vi "init.vi"(0 "Digital Input Test in":refnum<class "Set Motor Power Test.lvclass">, 1 "Command":u16, 2 "ConfigureILCStrategy":refnum<class "IConfigureILCStrategy.lvclass">, 5 "error in (no error)":errorcluster, 6 "Test Scenario":T1, 7 "Log":refnum<class "ITestLog.lvclass">, 8 "Signal Name":string) -> (14 "Digital Input Test out":refnum<class "Set Motor Power Test.lvclass">, 19 "error out":errorcluster)   [LabVIEW 2015, in "Set Motor Power Test.lvclass"]
uses:
  Set Motor Power Test.lvclass
  Model/TestLog/ITestLog/ITestLog.lvclass
  Typedefs/TestScenarioTypes.ctl
  Model/ConfigureILCStrategy/IConfigureILCStrategy/IConfigureILCStrategy.lvclass
  Set Motor Power Test.lvclass/Set Motor Power Test.ctl
  Typedefs/ILCBTTypedefs.lvlib
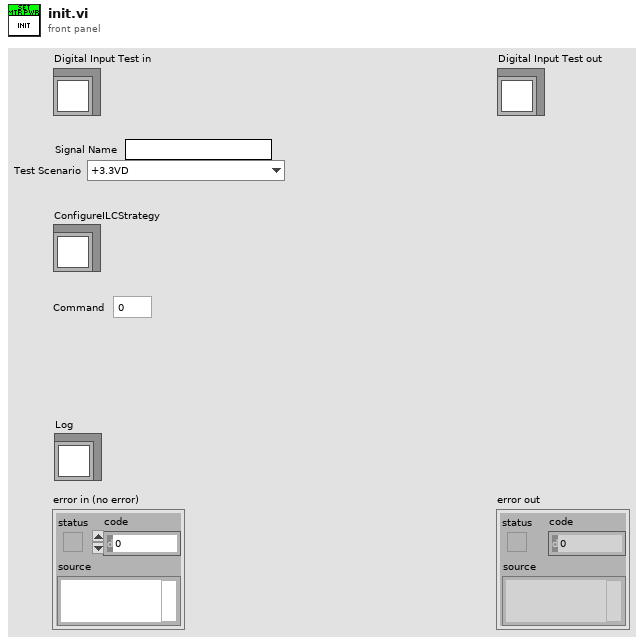
[diagram p1: front panel]
types:
  T1 = typedef "ILCBTTypedefs.lvlib/TestScenarioTypes.ctl" = enum16{"+3.3VD", "+5.1V", "+24V", "RELVALV1", "RELVALV2", "Verify DAC_A = -1.00A", "Verify DAC_A = -0.75A", "Verify DAC_A = -0.50A", "Verify DAC_A = -0.25A", "Verify DAC_A = 0.00A", "Verify DAC_A = 0.25A", "Verify DAC_A = 0.50A", "Verify DAC_A = 0.75A", "Verify DAC_A = 1.00A", "Verify DAC_B = -1.00A", "Verify DAC_B = -0.75A", "Verify DAC_B = -0.50A", "Verify DAC_B = -0.25A", "Verify DAC_B = 0.00A", "Verify DAC_B = 0.25A", "Verify DAC_B = 0.50A", "Verify DAC_B = 0.75A", "Verify DAC_B = 1.00A", "Set DAC_A = -1.00A", "Set DAC_A = -0.75A", "Set DAC_A = -0.50A", "Set DAC_A = -0.25A", "Set DAC_A = 0.00A", "Set DAC_A = 0.25A", "Set DAC_A = 0.50A", "Set DAC_A = 0.75A", "Set DAC_A = 1.00A", "Set DAC_B = -1.00A", "Set DAC_B = -0.75A", "Set DAC_B = -0.50A", "Set DAC_B = -0.25A", "Set DAC_B = 0.00A", "Set DAC_B = 0.25A", "Set DAC_B = 0.50A", "Set DAC_B = 0.75A", "Set DAC_B = 1.00A", "Set MTR_PWR = On", "Set MTR_PWR = Off"}
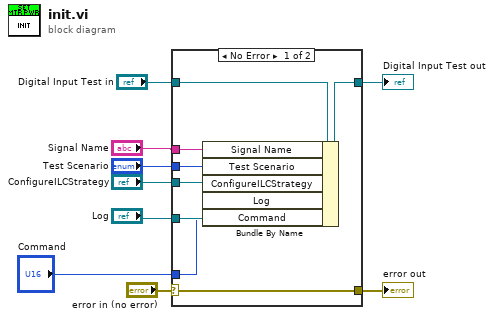
[diagram p0: block diagram]
diagram:
  n1 = case shown="No Error" "error in (no error)" {
    selector: "error in (no error)" -> [w17 w19]
    tunnel: [w17 w19] -> w8
    tunnel: [w13 w18] -> w6
    tunnel: "Digital Input Test in" -> [w16 w18]
    tunnel: "Signal Name" -> [w12 _]
    tunnel: "Test Scenario" -> [w11 _]
    tunnel: "ConfigureILCStrategy" -> [w14 _]
    tunnel: "Log" -> [w15 _]
    tunnel: "Command" -> [w10 _]
    frame No Error {
      n2 = Bundle By Name(cluster=w16, "Signal Name"=w12, "Test Scenario"=w11, "ConfigureILCStrategy"=w14, "Log"=w15, "Command"=w10) -> (w13:refnum<class "Set Motor Power Test.lvclass">)
    }
    frame Error {
    }
  }
  "error out" <- w8
  "Digital Input Test out" <- w6
